vi "Process.vi"(8 "error in":errorcluster, 11 "Example Instrument UI":refnum<class "ExampleInstrument.UI.lvclass">) -> (0 "error out":errorcluster, 3 "Example Instrument UI out":refnum<class "ExampleInstrument.UI.lvclass">)   [LabVIEW 2016, in "ExampleInstrument.UI.lvclass"]
doc: "---------------------------------------------------------------\nJKI State Machine Objects™\nhttp://jki.net/state-machine-objects/\nCopyright (C) 2005-2015, JKI <info@jki.net>\nALL RIGHTS RESERVEDJKI State Machine Objects (SMO) 1.0.0.5\nJKI - JKI\nCopyright (c) 2016, JKI"
uses:
  ExampleInstrument.UI.lvclass
  C:/Program Files (x86)/National Instruments/LabVIEW 2016/vi.lib/JKI/JKI SMO/SMO/SMO.lvclass
  C:/Program Files (x86)/National Instruments/LabVIEW 2016/vi.lib/JKI/JKI SMO/SMO.UI/SMO.UI.lvclass
  <vilib>/JKI/JKI SMO/SMO/Typedefs/Parent Call--Enum.ctl
  ExampleInstrument.UI.lvclass/ExampleInstrument.UI.ctl
  Example Instrument/Typedefs/ExampleInstrument.getAll--Cluster.ctl
  <vilib>/JKI/JKI SMO/SMO.UI/SMO.UI.lvclass
  lvsrc/SMOs/Instrument/Instrument.lvclass
  <vilib>/JKI/JKI SMO/SMO/SMO.lvclass
  Example Instrument/ExampleInstrument.lvclass
panel:
  out "Numeric":u32
  out "Instrument Response":dbl
  in  "Set Parameter":bool
  in  "Parameter":dbl
  in  "STOP":bool
  out "SMO string":string
  out "SMO Boolean":bool
  out "Logger SMO":dbl
  out "Levy 1":dbl
  # "#todo\nmake UI here. maybe include a nice picture of the hardware?"
  # "#todo\nadd buttons to do stuff (e.g., change a setting)\nButtons should trigger an event"
  # "#todo\nresize this box if you want your UI to be different size"
  # "SMO UI Template"
  # "For instructions on how to use the JKI State Machine Objects, examples and video tutorials, visit:\nhttp://jki.net/state-machine-objects/\n\nJKI State Machine Objects™\nhttp://jki.net/state-machine-objects/\nCopyright (C) 2005-2015, JKI <info@jki.net>\nALL RIGHTS RESERVED"
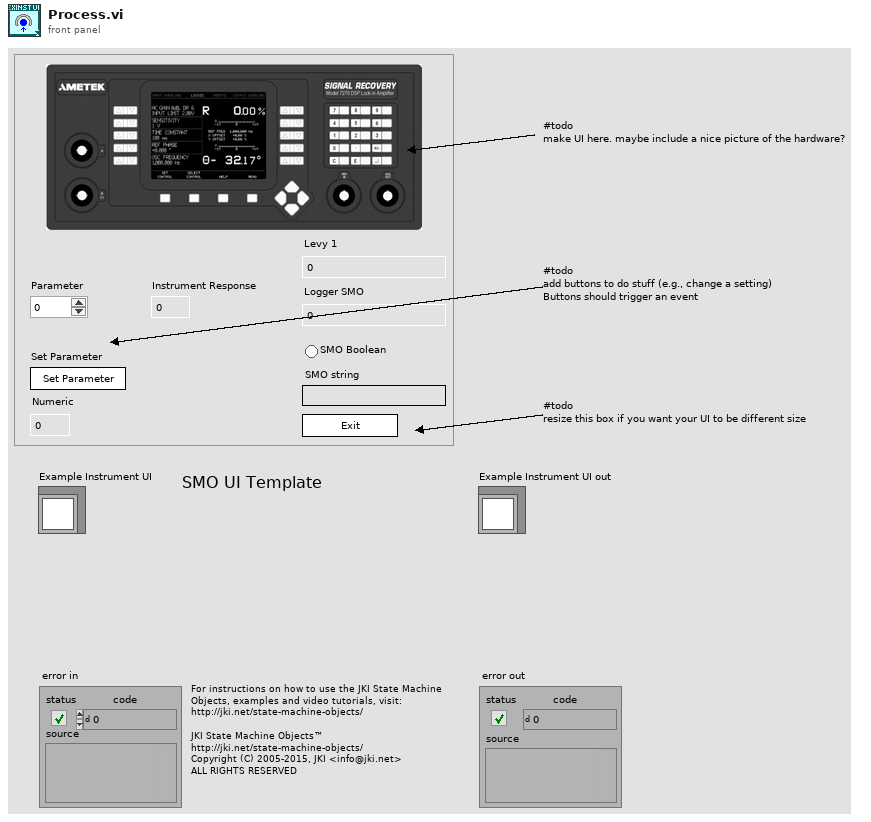
[diagram p1: front panel]
types:
  T1 = typedef "SMO.lvclass/Parent Call--Enum.ctl" = enum16{"Allows parent to run", "Does not request parent to run"}
  T2 = enum32{"invalid app kind", "Development System", "Run Time System", "Student Edition", "Embedded LabVIEW", "Evaluation", "Custom"}
  T3 = enum32{"Invalid", "Standard", "Closed", "Hidden", "Minimized", "Maximized"}
  T4 = typedef "ExampleInstrument.lvclass/ExampleInstrument.getAll--Cluster.ctl" = cluster{"Levy 1":dbl, "Logger SMO":dbl, "SMO Boolean":bool, "SMO String":string}
  T5 = cluster{"Core":cluster{"Current VI Reference":refnum<vi>, "Close Panel on Exit?":bool, "error":errorcluster}, "Self Reference":refnum<class "ExampleInstrument.UI.lvclass">, "Instrument":refnum<class "Instrument.lvclass">, "getAll":variant, "Parameter":dbl}
  T6 = cluster{"Current VI Reference":refnum<vi>, "Close Panel on Exit?":bool, "error":errorcluster}
  T7 = typedef "SMO.lvclass/Protected Events.ctl" = cluster{"StopProcesses":refnum<user-event>, "AbortProcesses":refnum<user-event>, "Config Changed":refnum<user-event>, "Dependency":refnum<user-event>}
  T8 = typedef "Instrument.lvclass/PublicEvents--Cluster.ctl" = cluster{"MessageFromProcess":refnum<user-event>}
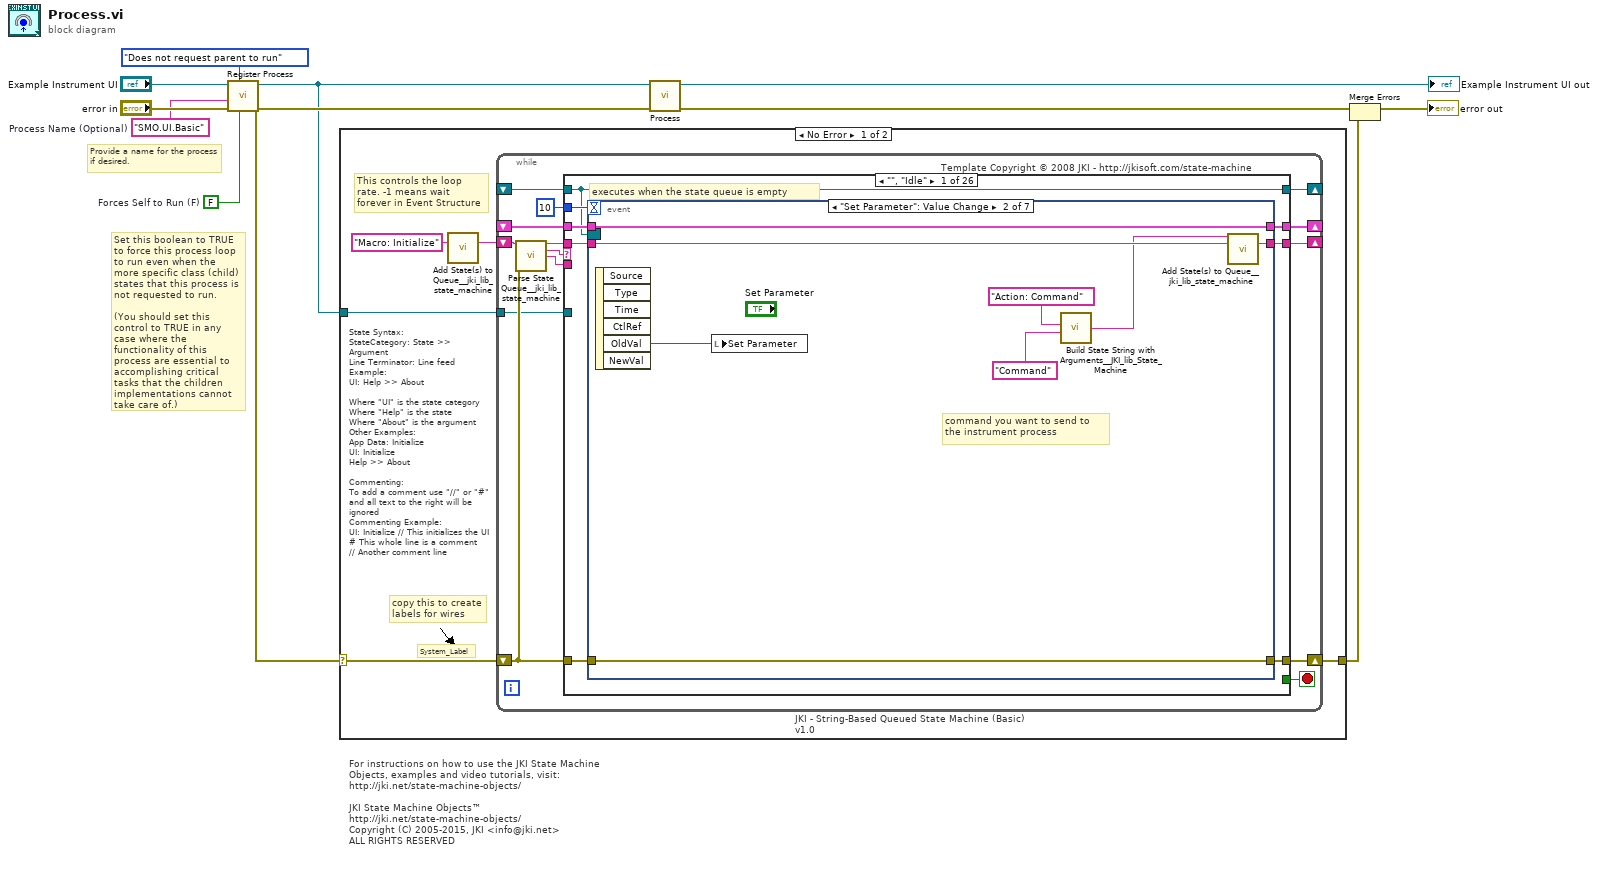
[diagram p0: block diagram]
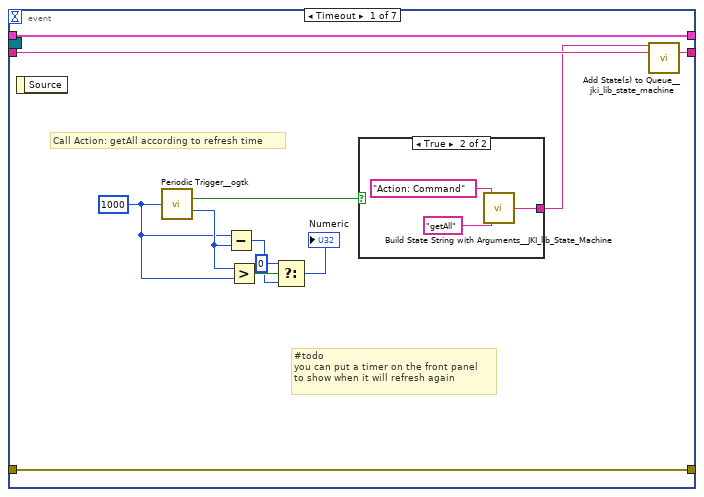
[diagram p2: hidden frame]
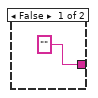
[diagram p3: hidden frame]
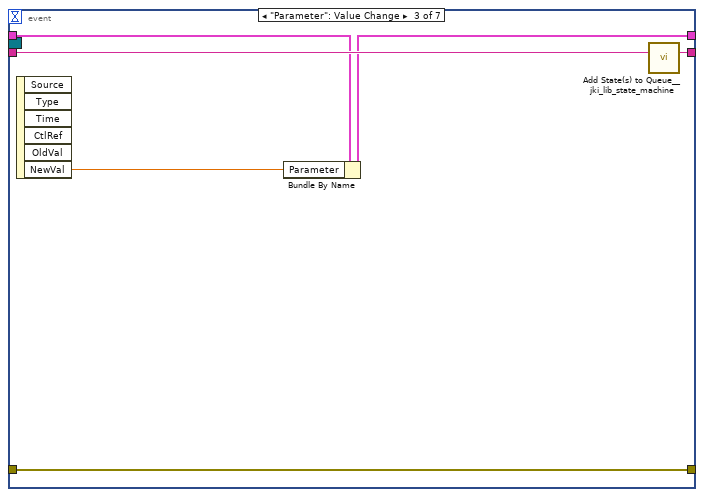
[diagram p4: hidden frame]
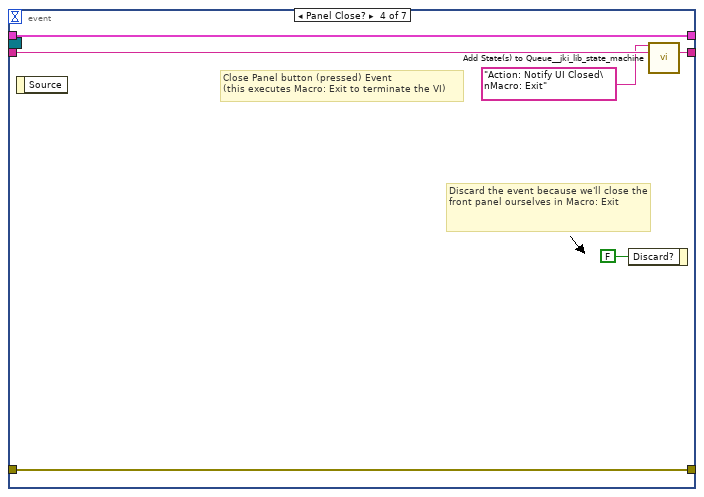
[diagram p5: hidden frame]
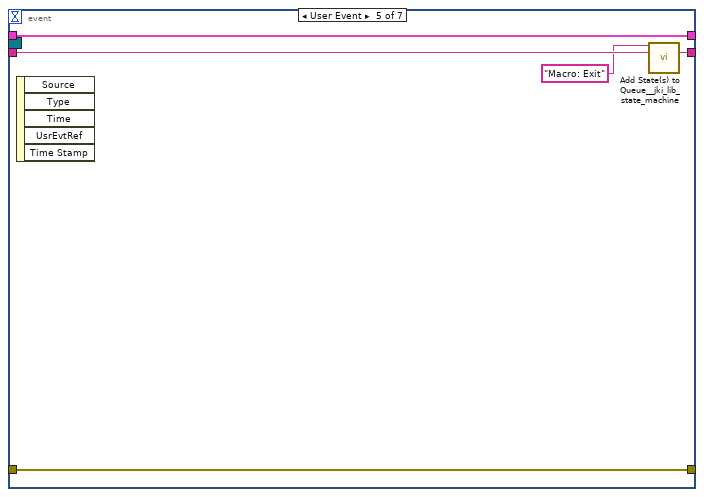
[diagram p6: hidden frame]
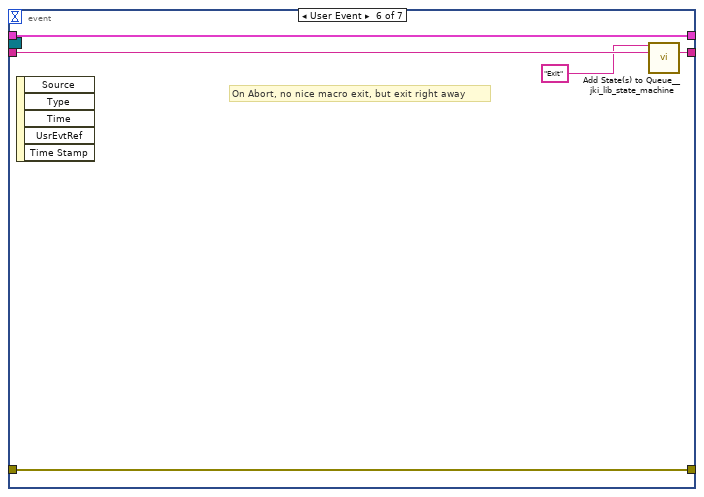
[diagram p7: hidden frame]
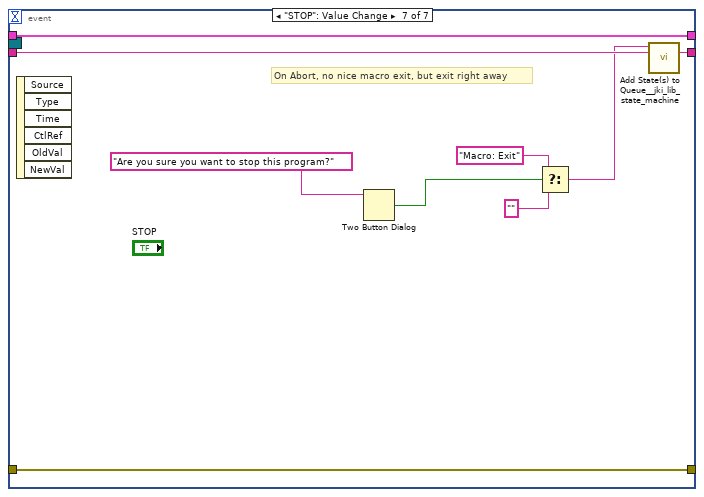
[diagram p8: hidden frame]
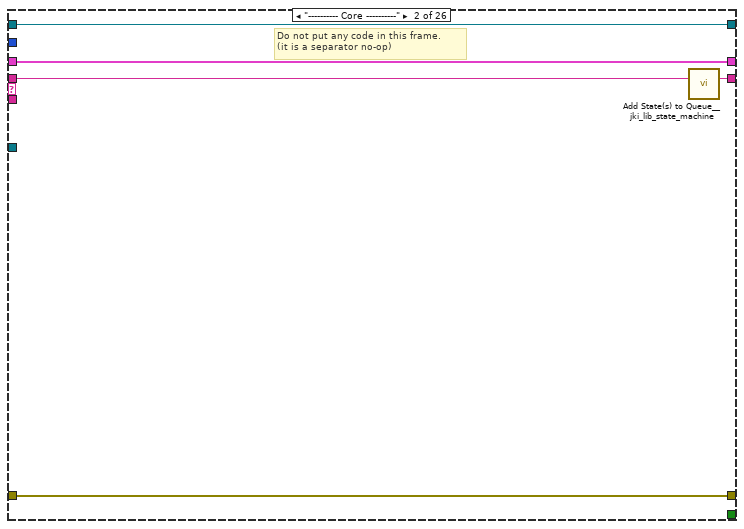
[diagram p9: hidden frame]
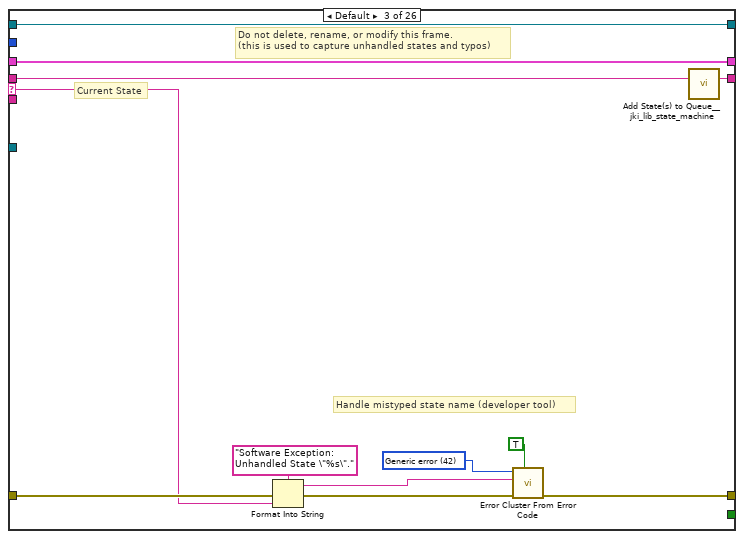
[diagram p10: hidden frame]
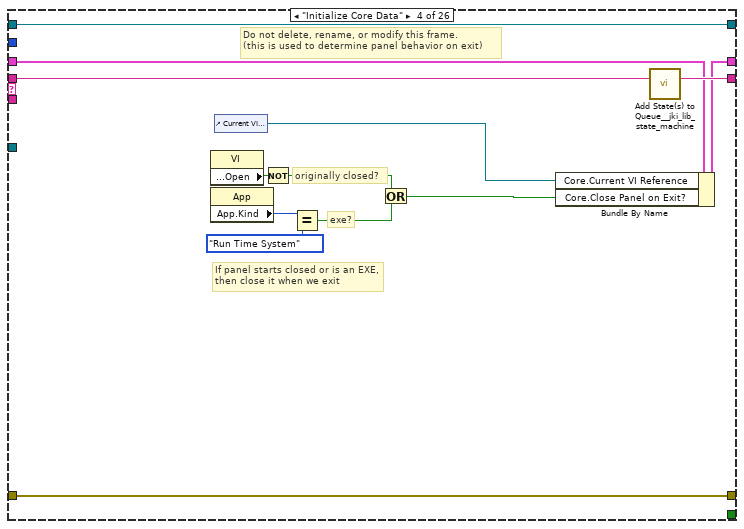
[diagram p11: hidden frame]
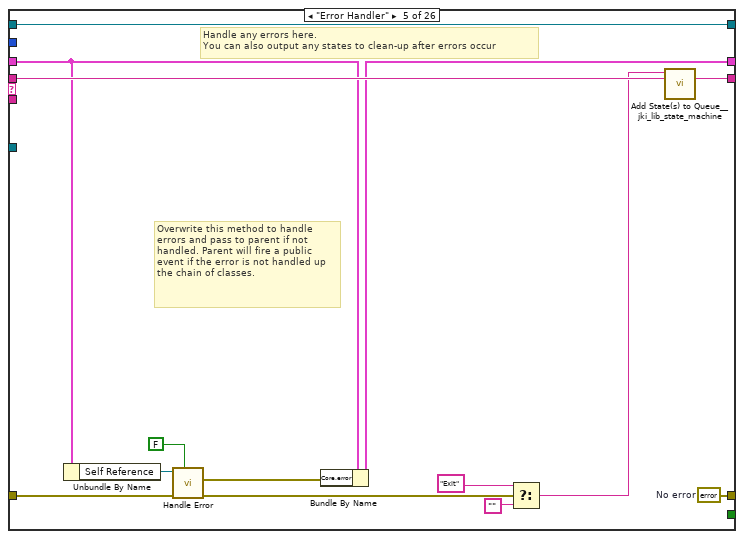
[diagram p12: hidden frame]
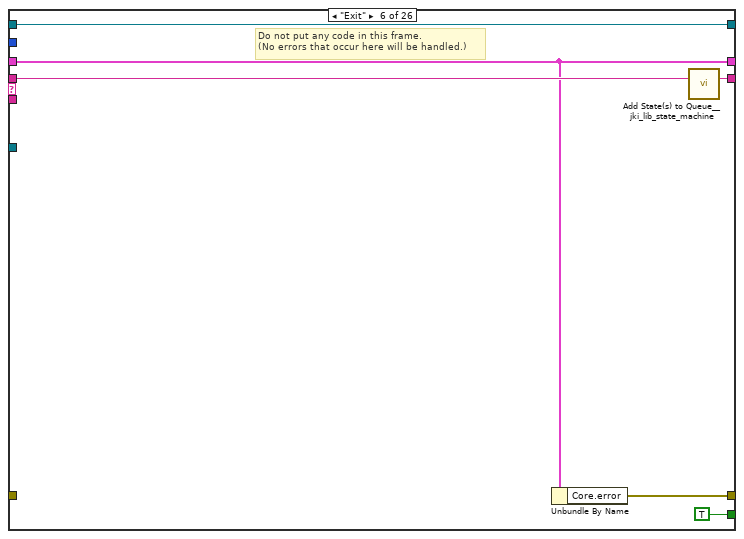
[diagram p13: hidden frame]
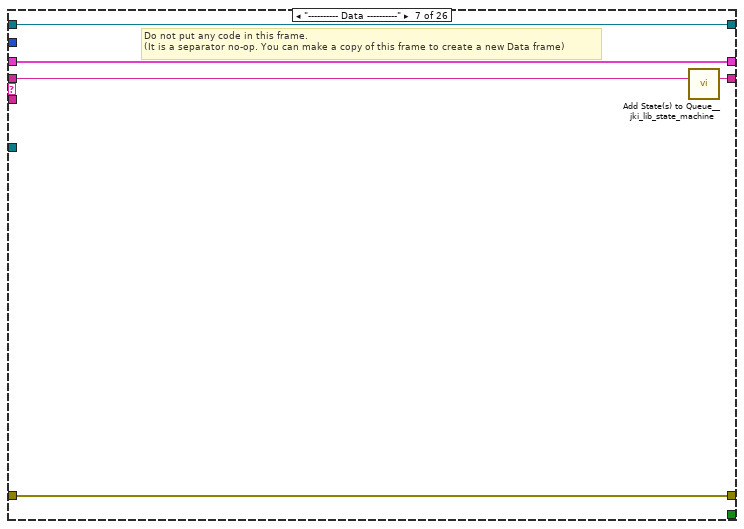
[diagram p14: hidden frame]
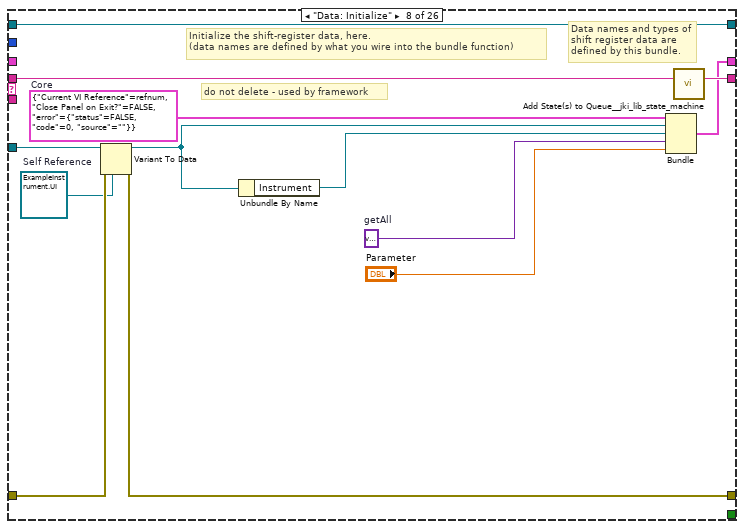
[diagram p15: hidden frame]
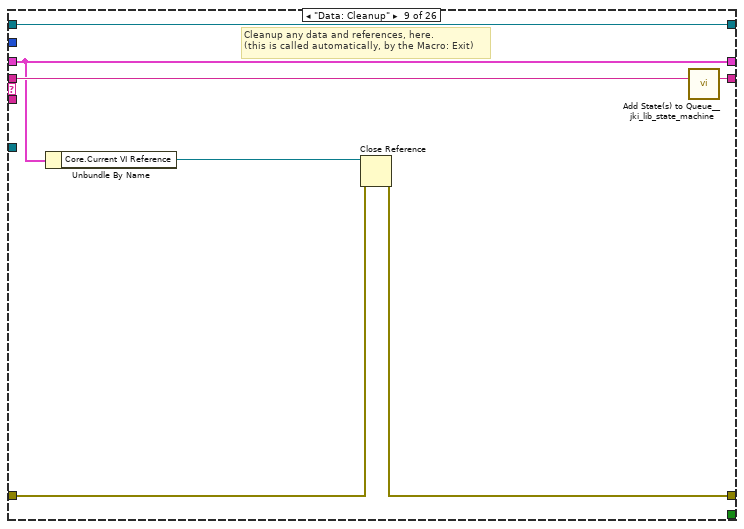
[diagram p16: hidden frame]
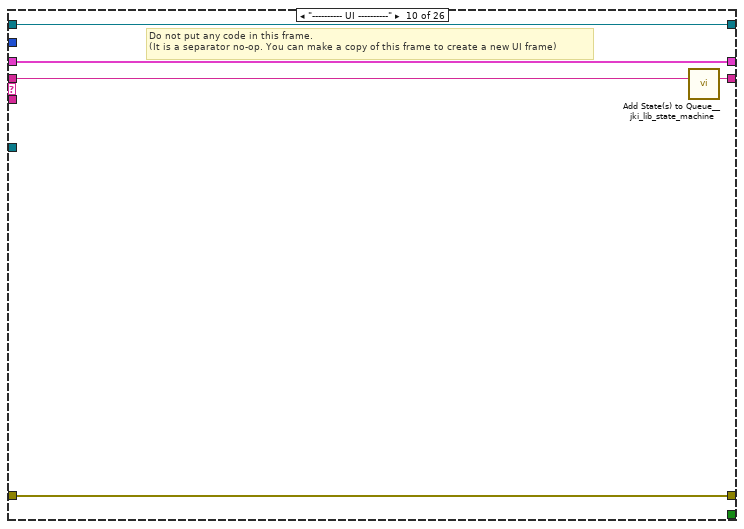
[diagram p17: hidden frame]
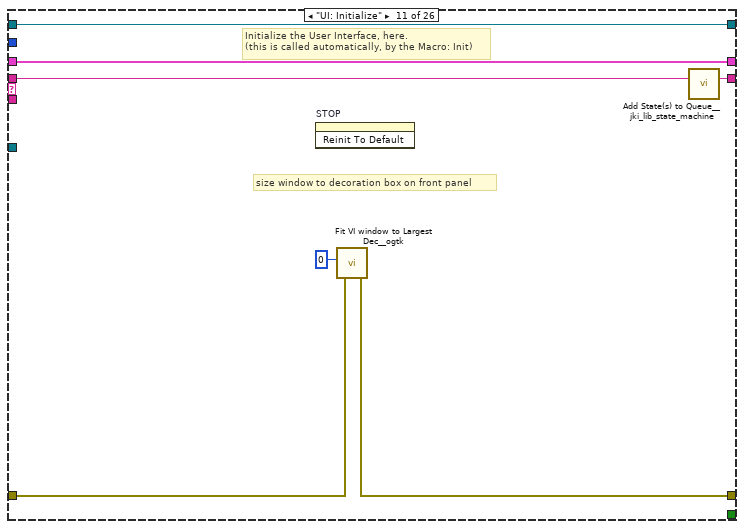
[diagram p18: hidden frame]
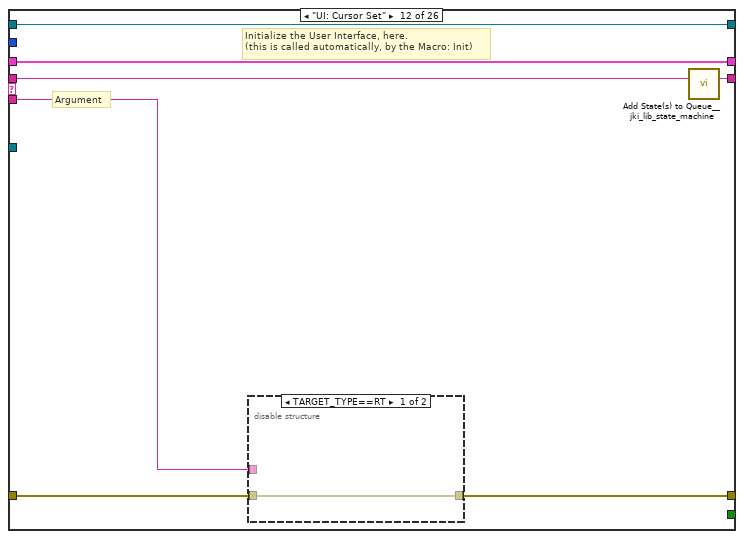
[diagram p19: hidden frame]
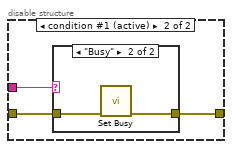
[diagram p20: hidden frame]
diagram:
  w2 = FALSE  # Forces Self to Run (F)
  w1 = "SMO.UI.Basic"  # Process Name (Optional)
  # "Provide a name for the process\nif desired."
  # "Set this boolean to TRUE to force this process loop to run even when the more specific class (child) states that this process is not requested to run.\n\n(You should set this control to TRUE in any case where the functionality of this process are essential to accomplishing critical tasks that the children implementations cannot take care of.)"
  # "For instructions on how to use the JKI State Machine Objects, examples and video tutorials, visit:\nhttp://jki.net/state-machine-objects/\n\nJKI State Machine Objects™\nhttp://jki.net/state-machine-objects/\nCopyright (C) 2005-2015, JKI <info@jki.net>\nALL RIGHTS RESERVED"
  n1 = call <vilib>:"Register Process.vi"("Forces Self to Run (F)"=w2, "Parent Call"=Parent_Call--Enum."Does not request parent to run", "error in (no error)"="error in", "Process Name (optional)"=w1, "SMO"="Example Instrument UI") -> ("error out"=w8:errorcluster, "SMO out"=w7:refnum<class "ExampleInstrument.UI.lvclass">)  [unwired: 5 in]
  n2 = case shown="No Error" w8 {
    selector: w8 -> [w13 w371]
    tunnel: w7 -> [w14 _]
    tunnel: [w12 w371] -> w4
    frame No Error {
      # "State Syntax:\nStateCategory: State >> Argument\nLine Terminator: Line feed\nExample:\nUI: Help >> About\n\nWhere \"UI\" is the state category\nWhere \"Help\" is the state\nWhere \"About\" is the argument\nOther Examples:\nApp Data: Initialize\nUI: Initialize\nHelp >> About\n\nCommenting:\nTo add a comment use \"//\" or \"#\" and all text to the right will be ignored\nCommenting Example:\nUI: Initialize // This initializes the UI\n# This whole line is a comment\n// Another comment line"
      # "copy this to create labels for wires"
      # "This controls the loop rate. -1 means wait forever in Event Structure"
      # "System_Label"
      n3 = call <vilib>:"Add State(s) to Queue__jki_lib_state_machine.vi"("State(s) in (\"\")"="Macro: Initialize") -> ("States Out"=w16:string)  [unwired: 14 in]
      n4 = while "JKI - String-Based Queued State Machine (Basic) v1.0" {
        shift-right: [w23] -> _
        shift-left: _ -> [w22]
        shift-right: [w26] -> w12
        shift-left: w13 -> [w20]
        shift-right: [w25] -> _
        shift-left: w16 -> [w27]
        tunnel: w14 -> [w19]
        shift-right: [w18] -> _
        shift-left: _ -> [w17]
        stop <- w24 stop-if-true
        # "Template Copyright © 2008 JKI - http://jkisoft.com/state-machine"
        n5 = call <vilib>:"Parse State Queue__jki_lib_state_machine.vi"("State Queue"=w27, "Error In (no error)"=w20) -> ("Remaining States"=w29:string, "Current State"=w30:string, "Arguments"=w28:string)  [unwired: 11 in]
        n6 = case shown="\"\", \"Idle\"" w30 {
          selector: w30 -> [_ _ w100 _ _ _ _ _ _ _ _ _ _ _ _ _ _ _ _ _ _ _ _ _ _ _]
          tunnel: w29 -> [w38 w98 w104 w123 w137 w143 w148 w161 w168 w173 w180 w187 w203 w235 w244 w258 w263 w274 w281 w286 w299 w305 w312 w319 w332 w351]
          tunnel: w28 -> [_ _ _ _ _ _ _ _ _ _ _ w181 w197 _ _ _ _ _ _ _ _ _ _ _ _ w339]
          tunnel: w22 -> [w36 w95 w102 w114 w126 w139 w145 _ w163 w170 w178 w185 w199 w232 w240 w249 w260 w271 w276 w283 w297 w303 w308 w315 w329 w348]
          tunnel: [w35 w96 w106 w120 w128 w138 w146 w157 w164 w171 w175 w182 w200 w233 w242 w256 w261 w265 w277 w284 w292 w300 w309 w313 w325 w341] -> w26
          tunnel: w20 -> [w34 w96 w105 w120 w133 _ w146 w158 w165 w171 w176 w183 w201 w233 w242 w256 w261 w266 w278 w284 w294 w301 w309 w314 w326 w342]
          tunnel: [w37 w97 w103 w122 w136 w142 w147 w160 w167 w172 w179 w186 w202 w234 w243 w257 w262 w273 w280 w285 w298 w304 w311 w318 w331 w350] -> w25
          tunnel: [_ _ _ _ _ TRUE _ _ _ _ _ _ _ _ _ _ _ _ _ _ _ _ _ _ _ _] -> w24
          tunnel: [w33 w95 w102 w121 w125 w139 w145 w159 w163 w170 w178 w185 w199 w232 w240 w249 w260 w271 w276 w283 w297 w303 w307 w315 w329 w345] -> w23
          tunnel: 10 ("Timeout") -> [w32 _ _ _ _ _ _ _ _ _ _ _ _ _ _ _ _ _ _ _ _ _ _ _ _ _]
          tunnel: w19 -> [_ _ _ _ _ _ _ w155 _ _ _ _ _ _ _ _ _ _ _ _ _ _ _ _ _ _]
          tunnel: [w31 w94 w99 w111 w135 w140 w144 w154 w162 w169 w177 w184 w196 w231 w241 w250 w259 w272 w279 w282 w296 w302 w310 w317 w330 w349] -> w18
          tunnel: w17 -> [w31 w94 w99 w111 w135 w140 w144 w154 w162 w169 w177 w184 w196 w231 w241 w250 w259 w272 w279 w282 _ w302 w310 w317 w330 w349]
          frame "", "Idle" {
            # "executes when the state queue is empty"
            n7 = event shown="[1] \"Set Parameter\": Value Change" {
              selector: w31 -> [_ _ _ _ _ _ _]
              dyn-events: _ -> [_ _ _ _ _ _ _]
              timeout: w32 -> [_ _ _ _ _ _ _]
              tunnel: w38 -> [w50 w62 w68 w74 w79 w84 w93]
              tunnel: [w49 w61 w67 w73 w78 w83 w92] -> w37
              tunnel: w36 -> [w47 w59 w64 w70 w76 w81 w90]
              tunnel: [w48 w60 w66 w69 w77 w82 w91] -> w35
              tunnel: w34 -> [w48 w60 w66 w69 w77 w82 w91]
              tunnel: [w47 w59 w63 w70 w76 w81 w90] -> w33
              event Timeout {
                w43 = u32 1000 ("time (ms)")
                # "#todo\nyou can put a timer on the front panel\nto show when it will refresh again"
                # "Call Action: getAll according to refresh time"
                n8 = event-data() -> ()  [unwired: 1 in, 1 out]
                n9 = call <userlib>:"Periodic Trigger__ogtk.vi"("time (ms)"=w43) -> ("Triggered"=w45:bool, "timer value"=w44:u32)  [unwired: 12 in, 1 out]
                n10 = Subtract(x=w43, y=w44) -> (x-y=w40:u32)
                n11 = Greater?(x=w44, y=w43) -> (0:w42:bool)
                n12 = Select(t=u32 0, s=w42, f=w40) -> (s? t:f=→"Numeric":u32)
                n13 = case shown="True" w45 {
                  tunnel: ["" ("State(s) in Front (\"\")") w52] -> w46
                  frame False {
                  }
                  frame True {
                    n14 = call <vilib>:"Build State String with Arguments__JKI_lib_State_Machine.vi"("Arguments (\"\")"="getAll" ("State(s) in Front (\"\")"), "State"="Action: Command" ("State(s) in Front (\"\")")) -> ("State with Arguments"=w52:string)  [unwired: 4 in]
                  }
                }
                n15 = call <vilib>:"Add State(s) to Queue__jki_lib_state_machine.vi"("State(s) in Front (\"\")"=w46, "State(s) in (\"\")"=w50) -> ("States Out"=w49:string)  [unwired: 13 in]
              }
              event "Set Parameter": Value Change {
                # "command you want to send to\nthe instrument process"
                n16 = event-data() -> ("OldVal"=w58:bool)  [unwired: 1 in, 5 out]
                n17 = local write "Set Parameter"(w58) -> ()
                n18 = call <vilib>:"Build State String with Arguments__JKI_lib_State_Machine.vi"("Arguments (\"\")"="Command" ("State(s) in Front (\"\")"), "State"="Action: Command" ("State(s) in Front (\"\")")) -> ("State with Arguments"=w55:string)  [unwired: 4 in]
                n19 = call <vilib>:"Add State(s) to Queue__jki_lib_state_machine.vi"("State(s) in Front (\"\")"=w55, "State(s) in (\"\")"=w62) -> ("States Out"=w61:string)  [unwired: 13 in]
              }
              event "Parameter": Value Change {
                n20 = event-data() -> ("NewVal"=w65:dbl)  [unwired: 1 in, 5 out]
                n21 = Bundle By Name(cluster=w64, "Parameter"=w65) -> (w63:T5)
                n22 = call <vilib>:"Add State(s) to Queue__jki_lib_state_machine.vi"("State(s) in (\"\")"=w68) -> ("States Out"=w67:string)  [unwired: 14 in]
              }
              event Panel Close? {
                # "Discard the event because we'll close the front panel ourselves in Macro: Exit"
                # "Close Panel button (pressed) Event\n(this executes Macro: Exit to terminate the VI)"
                n23 = event-data() -> ()  [unwired: 1 in, 1 out]
                n24 = event-data("Discard?"=FALSE) -> ()  [unwired: 1 in, 1 out]
                n25 = call <vilib>:"Add State(s) to Queue__jki_lib_state_machine.vi"("State(s) in Front (\"\")"="Action: Notify UI Closed\nMacro: Exit", "State(s) in (\"\")"=w74) -> ("States Out"=w73:string)  [unwired: 13 in]
              }
              event User Event {
                n26 = event-data() -> ()  [unwired: 1 in, 5 out]
                n27 = call <vilib>:"Add State(s) to Queue__jki_lib_state_machine.vi"("State(s) in Front (\"\")"="Macro: Exit", "State(s) in (\"\")"=w79) -> ("States Out"=w78:string)  [unwired: 13 in]
              }
              event User Event {
                # "On Abort, no nice macro exit, but exit right away"
                n28 = event-data() -> ()  [unwired: 1 in, 5 out]
                n29 = call <vilib>:"Add State(s) to Queue__jki_lib_state_machine.vi"("State(s) in Front (\"\")"="Exit", "State(s) in (\"\")"=w84) -> ("States Out"=w83:string)  [unwired: 13 in]
              }
              event "STOP": Value Change {
                # "On Abort, no nice macro exit, but exit right away"
                n30 = event-data() -> ()  [unwired: 1 in, 6 out]
                n31 = Two Button Dialog(message="Are you sure you want to stop this program?") -> (T button?=w89:bool)  [unwired: 2 in]
                n32 = Select(t="Macro: Exit", s=w89, f="") -> (s? t:f=w85:string)
                n33 = call <vilib>:"Add State(s) to Queue__jki_lib_state_machine.vi"("State(s) in Front (\"\")"=w85, "State(s) in (\"\")"=w93) -> ("States Out"=w92:string)  [unwired: 13 in]
              }
            }
          }
          frame "---------- Core ----------" {
            # "Do not put any code in this frame.\n(it is a separator no-op)"
            n34 = call <vilib>:"Add State(s) to Queue__jki_lib_state_machine.vi"("State(s) in (\"\")"=w98) -> ("States Out"=w97:string)  [unwired: 14 in]
          }
          frame Default {
            w109 = 42 items=["No error", "Argument error", "Memory is full", "Out of zone", "End of file", "File already open", "Generic file I/O error", "File not found", "File permission error", "Disk is full", "Duplicate path", "Too many files open", "System feature not enabled", "Resource file not found", "Cannot add resource", "Resource not found", "Image not found", "Image memory error", "Pen does not exist", "Config type invalid", "Config token not found", "Config parse error", "Config memory error", "Bad external code format", "Bad external code offset", "External code not present", "Null window", "Destroy window error", "Null menu", "Print aborted", "Bad print record", "Print driver error", "Windows error during printing", "Memory error during printing", "Print dialog error", "Generic print error", "Invalid device refnum", "Device not found", "Device parameter error", "Device unit error", "Cannot open device", "Device call aborted", "Generic error", "Cancelled by user", "Object ID too low", "Object ID too high", "Object not in heap", "Unknown heap", "Unknown object (invalid DefProc)", "Unknown object (DefProc not in table)", "Message out of range", "Invalid (null) method", "Unknown message", "Manager call not supported", "Bad address", "Network operation in progress", "Network operation timed out", "Connection is busy", "Network attribute not supported", "Network error", "Address in use", "System out of memory", "Connection aborted", "Connection refused", "Not connected", "Already connected", "Connection closed", "Initialization error (interapplication manager)", "Bad occurrence", "Wait on unbound occurrence handler", "Occurrence queue overflow", "Datalog type conflict", "Unused", "Unrecognized type (interapplication manager)", "Memory corrupt", "Failed to make temporary DLL", "Old CIN version", "Drag socket not found", "Failed to load drop-object", "Failed to register OLE object", "Failed to release OLE object", "Format specifier type mismatch", "Unknown format specifier", "Too few format specifiers", "Too many format specifiers", "Scan failed", "Newer CIN version", "Error converting to variant", "Runtime menu error", "Password tampered", "Variant attribute not found", "Incompatible variant data type", "Event data is not available", "Event Store is not present", "Occurrence is not found", "Event Queue is not created", "Event info is not available", "Refnum passed is NULL", "Error retrieving Class GUID", "Error retrieving CoClass GUID", "Error retrieving TypeLib GUID.", "Bad built application magic bytes.", "Specific driver is different from the specific driver associated with the Logical Name.", "There is no session opened to the class driver.", "Max Error", "MAX - Error with config objects", "MAX - Error loading configuration", "MAX - Group not supported"]
            # "Current State"
            # "Do not delete, rename, or modify this frame.\n(this is used to capture unhandled states and typos)"
            # "Handle mistyped state name (developer tool)"
            n35 = Format Into String(format string="Software Exception: Unhandled State \"%s\"." ("message"), error in=w105, w100) -> (resulting string=w108:string, error out=w107:errorcluster)  [unwired: 1 in]
            n36 = call <vilib>:"Error Cluster From Error Code.vi"("show call chain? (False)"=TRUE, "error in (no error)"=w107, "error message (\"\")"=w108, "error code (0)"=w109) -> ("error out"=w106:errorcluster)  [unwired: 5 in]
            n37 = call <vilib>:"Add State(s) to Queue__jki_lib_state_machine.vi"("State(s) in (\"\")"=w104) -> ("States Out"=w103:string)  [unwired: 14 in]
          }
          frame "Initialize Core Data" {
            # "Do not delete, rename, or modify this frame.\n(this is used to determine panel behavior on exit)"
            # "originally closed?"
            # "exe?"
            # "If panel starts closed or is an EXE, then close it when we exit"
            n38 = property class="VI"() -> ("Front Panel.Open"=w119:bool)  [unwired: 2 in, 2 out]
            n39 = property class="App"() -> ("App.Kind"=w118:T2)  [unwired: 2 in, 2 out]
            n40 = control-ref of="Current VI Reference"() -> (w112:refnum<vi>)
            n41 = Not(x=w119) -> (.not. x?=w116:bool)
            n42 = Equal?(x=w118, y=T2."Run Time System" ("Application:Kind")) -> (x = y?=w115:bool)
            n43 = Or(x=w116, y=w115) -> (x .or. y?=w113:bool)
            n44 = Bundle By Name(cluster=w114, "Core.Current VI Reference"=w112, "Core.Close Panel on Exit?"=w113) -> (w121:T5)
            n45 = call <vilib>:"Add State(s) to Queue__jki_lib_state_machine.vi"("State(s) in (\"\")"=w123) -> ("States Out"=w122:string)  [unwired: 14 in]
          }
          frame "Error Handler" {
            w128 = errorcluster {"status"=FALSE, "code"=0, "source"=""}  # No error
            # "Overwrite this method to handle errors and pass to parent if not handled. Parent will fire a public event if the error is not handled up the chain of classes."
            # "Handle any errors here.\nYou can also output any states to clean-up after errors occur"
            n46 = Unbundle By Name(w126) -> ("Self Reference"=w134:refnum<class "ExampleInstrument.UI.lvclass">)
            n47 = call-dynamic "Handle Error.vi"("Stop on Unhandled Error (T)"=FALSE, "error in"=w133, "SMO"=w134) -> ("handling error"=w129:errorcluster, "Unhandled error"=w127:errorcluster)  [unwired: 6 in, 1 out]
            n48 = Bundle By Name(cluster=w126, "Core.error"=w127) -> (w125:T5)
            n49 = Select(t="Exit", s=w129, f="") -> (s? t:f=w130:string)
            n50 = call <vilib>:"Add State(s) to Queue__jki_lib_state_machine.vi"("State(s) in Front (\"\")"=w130, "State(s) in (\"\")"=w137) -> ("States Out"=w136:string)  [unwired: 13 in]
          }
          frame "Exit" {
            # "Do not put any code in this frame.\n(No errors that occur here will be handled.)"
            n51 = Unbundle By Name(w139) -> ("Core.error"=w138:errorcluster)
            n52 = call <vilib>:"Add State(s) to Queue__jki_lib_state_machine.vi"("State(s) in (\"\")"=w143) -> ("States Out"=w142:string)  [unwired: 14 in]
          }
          frame "---------- Data ----------" {
            # "Do not put any code in this frame.\n(It is a separator no-op. You can make a copy of this frame to create a new Data frame)"
            n53 = call <vilib>:"Add State(s) to Queue__jki_lib_state_machine.vi"("State(s) in (\"\")"=w148) -> ("States Out"=w147:string)  [unwired: 14 in]
          }
          frame "Data: Initialize" {
            w150 = variant  # getAll
            w153 = T6 {"Current VI Reference"=refnum, "Close Panel on Exit?"=FALSE, "error"={"status"=FALSE, "code"=0, "source"=""}}  # Core
            w156 = refnum<class "ExampleInstrument.UI.lvclass"> refnum  # Self Reference
            # "do not delete - used by framework"
            # "Data names and types of shift register data are defined by this bundle."
            # "Initialize the shift-register data, here.\n(data names are defined by what you wire into the bundle function)"
            n54 = Variant To Data(error in=w158, type=w156, Variant=w155) -> (data=w152:refnum<class "ExampleInstrument.UI.lvclass">, error out=w157:errorcluster)
            n55 = Unbundle By Name(w152) -> ("Instrument"=w151:refnum<class "Instrument.lvclass">)
            n56 = Bundle("Core"=w153, "Self Reference"=w152, "Instrument"=w151, "getAll"=w150, "Parameter"="Parameter") -> (w159:T5)  [unwired: 1 in]
            n57 = call <vilib>:"Add State(s) to Queue__jki_lib_state_machine.vi"("State(s) in (\"\")"=w161) -> ("States Out"=w160:string)  [unwired: 14 in]
          }
          frame "Data: Cleanup" {
            # "Cleanup any data and references, here.\n(this is called automatically, by the Macro: Exit)"
            n58 = Unbundle By Name(w163) -> ("Core.Current VI Reference"=w166:refnum<vi>)
            n59 = Close Reference(reference=w166, error in (no error)=w165) -> (error out=w164:errorcluster)
            n60 = call <vilib>:"Add State(s) to Queue__jki_lib_state_machine.vi"("State(s) in (\"\")"=w168) -> ("States Out"=w167:string)  [unwired: 14 in]
          }
          frame "---------- UI ----------" {
            # "Do not put any code in this frame.\n(It is a separator no-op. You can make a copy of this frame to create a new UI frame)"
            n61 = call <vilib>:"Add State(s) to Queue__jki_lib_state_machine.vi"("State(s) in (\"\")"=w173) -> ("States Out"=w172:string)  [unwired: 14 in]
          }
          frame "UI: Initialize" {
            # "size window to decoration box on front panel"
            # "Initialize the User Interface, here.\n(this is called automatically, by the Macro: Init)"
            n62 = invoke on="STOP" class="Bool (strict)" method="Reinit To Default"() -> ()  [unwired: 3 in, 3 out]
            n63 = call <userlib>:"Fit VI window to Largest Dec__ogtk.vi"("error in (no error)"=w176, "border spacing (2 px)"=0) -> ("error out"=w175:errorcluster)  [unwired: 4 in, 1 out]
            n64 = call <vilib>:"Add State(s) to Queue__jki_lib_state_machine.vi"("State(s) in (\"\")"=w180) -> ("States Out"=w179:string)  [unwired: 14 in]
          }
          frame "UI: Cursor Set" {
            # "Argument"
            # "Initialize the User Interface, here.\n(this is called automatically, by the Macro: Init)"
            n65 = disable-structure shown="TARGET_TYPE==RT" {
              disable-tunnel: w183 -> [w188 w191]
              disable-tunnel: [w188 w190] -> w182
              disable-tunnel: w181 -> [_ w189]
              frame condition #0 {
              }
              frame condition #1 (active) {
                n66 = case shown="\"Busy\"" w189 {
                  tunnel: w191 -> [w193 w195]
                  tunnel: [w192 w194] -> w190
                  frame "Idle", Default {
                    n67 = call <vilib>:"Unset Busy.vi"("error in (no error)"=w193) -> ("error out"=w192:errorcluster)  [unwired: 10 in]
                  }
                  frame "Busy" {
                    n68 = call <vilib>:"Set Busy.vi"("error in (no error)"=w195) -> ("error out"=w194:errorcluster)  [unwired: 9 in, 1 out]
                  }
                }
              }
            }
            n69 = call <vilib>:"Add State(s) to Queue__jki_lib_state_machine.vi"("State(s) in (\"\")"=w187) -> ("States Out"=w186:string)  [unwired: 14 in]
          }
          frame "UI: Front Panel State" {
            # "Argument"
            # "Set Front Panel Open or Closed\n(Usage: \"UI: Front Panel State >> Open|Close\")"
            n70 = Unbundle By Name(w199) -> ("Core.Current VI Reference"=w198:refnum<vi>)
            n71 = disable-structure shown="Default" {
              disable-tunnel: w201 -> [w207 w230]
              disable-tunnel: [w206 w230] -> w200
              disable-tunnel: w198 -> [w205 _]
              disable-tunnel: w197 -> [w204 _]
              frame condition #0 (active) {
                n72 = case shown="\"Close\"" w204 {
                  tunnel: w207 -> [w211 w224]
                  tunnel: [w213 w225] -> w206
                  tunnel: w205 -> [w212 w222]
                  frame "Open", Default {
                    n73 = property class="VI"(reference=w212, error in=w211) -> (reference out=w209:refnum<vi>, error out=w210:errorcluster, "FP.State"=w208:T3)
                    n74 = case shown="\"Closed\"" w208 {
                      tunnel: [w216 w219] -> w213
                      tunnel: w210 -> [w215 w219]
                      tunnel: w209 -> [w214 _]
                      frame "Closed" {
                        n75 = invoke class="VI" method="FP.Open"(reference=w214, error in=w215, "Activate"=TRUE, "State"=T3."Standard") -> (error out=w216:errorcluster)  [unwired: 1 in, 4 out]
                      }
                      frame Default {
                      }
                    }
                  }
                  frame "Close" {
                    n76 = property class="VI"(reference=w222, error in=w224) -> (reference out=w221:refnum<vi>, error out=w223:errorcluster, "FP.State"=w220:T3)
                    n77 = case shown="Default" w220 {
                      tunnel: [w226 w229] -> w225
                      tunnel: w223 -> [w226 w228]
                      tunnel: w221 -> [_ w227]
                      frame "Invalid", "Closed" {
                      }
                      frame Default {
                        n78 = invoke class="VI" method="FP.Close"(reference=w227, error in=w228) -> (error out=w229:errorcluster)  [unwired: 1 in, 2 out]
                      }
                    }
                  }
                }
              }
              frame condition #1 {
              }
            }
            n79 = call <vilib>:"Add State(s) to Queue__jki_lib_state_machine.vi"("State(s) in (\"\")"=w203) -> ("States Out"=w202:string)  [unwired: 14 in]
          }
          frame "---------- Macro ----------" {
            # "Do not put any code in this frame.\n(It is a separator no-op. You can make a copy of this frame to create a new Macro frame)"
            n80 = call <vilib>:"Add State(s) to Queue__jki_lib_state_machine.vi"("State(s) in (\"\")"=w235) -> ("States Out"=w234:string)  [unwired: 14 in]
          }
          frame "Macro: Initialize" {
            w238 = "UI: Initialize\n//UI: Front Panel State >> Open"  # UI: Initialize //UI: Front Panel State >> Open
            # "Initialization Macro\n(This is called once, when the VI starts)"
            n81 = call <vilib>:"Add State(s) to Queue__jki_lib_state_machine.vi"("State(s) in Front (\"\")"="Data: Initialize\nInitialize Core Data\nEvents: Register", "State(s) in (\"\")"="Process: Sync", "State(s) at Back (\"\")"=w238) -> ("States Out"=w237:string)  [unwired: 12 in]
            n82 = call <vilib>:"Add State(s) to Queue__jki_lib_state_machine.vi"("State(s) in Front (\"\")"=w237, "State(s) in (\"\")"=w244) -> ("States Out"=w243:string)  [unwired: 13 in]
          }
          frame "Macro: Exit" {
            # "Exit Macro\n(This is called once, when the VI exits)"
            n83 = Unbundle By Name(w249) -> ("Core.Close Panel on Exit?"=w255:bool)
            n84 = Select(t="//UI: Front Panel State >> Close", s=w255, f="") -> (s? t:f=w252:string)
            n85 = call <vilib>:"Add State(s) to Queue__jki_lib_state_machine.vi"("State(s) in Front (\"\")"="Data: Cleanup\nEvents: Unregister\nProcess: Self Terminate", "State(s) in (\"\")"="Process: Sync", "State(s) at Back (\"\")"="Exit") -> ("States Out"=w246:string)  [unwired: 12 in]
            n86 = call <vilib>:"Add State(s) to Queue__jki_lib_state_machine.vi"("State(s) in (\"\")"=w252, "State(s) at Back (\"\")"=w246) -> ("States Out"=w251:string)  [unwired: 13 in]
            n87 = call <vilib>:"Add State(s) to Queue__jki_lib_state_machine.vi"("State(s) in Front (\"\")"=w251, "State(s) in (\"\")"=w258) -> ("States Out"=w257:string)  [unwired: 13 in]
          }
          frame "---------- Process ----------" {
            # "Template Separator\n(You can make a copy of, or modify, this frame)"
            n88 = call <vilib>:"Add State(s) to Queue__jki_lib_state_machine.vi"("State(s) in (\"\")"=w263) -> ("States Out"=w262:string)  [unwired: 14 in]
          }
          frame "Process: Sync" {
            n89 = Unbundle By Name(w271) -> ("Self Reference"=w267:refnum<class "ExampleInstrument.UI.lvclass">)
            n90 = call <vilib>:"WaitOnProcessSync.vi"("error in (no error)"=w266, "SMO"=w267) -> ("error out"=w265:errorcluster, "Don't run?"=w270:bool)  [unwired: 7 in, 1 out]
            n91 = Select(t="Data: Cleanup\nEvents: Unregister\nExit", s=w270, f="") -> (s? t:f=w264:string)
            n92 = call <vilib>:"Add State(s) to Queue__jki_lib_state_machine.vi"("State(s) in Front (\"\")"=w264, "State(s) in (\"\")"=w274) -> ("States Out"=w273:string)  [unwired: 13 in]
          }
          frame "Process: Self Terminate" {
            n93 = Unbundle By Name(w276) -> ("Self Reference"=w275:refnum<class "ExampleInstrument.UI.lvclass">)
            n94 = call <vilib>:"SelfTerminate.vi"("error in (no error)"=w278, "SMO in"=w275) -> ("error out"=w277:errorcluster)  [unwired: 8 in, 1 out]
            n95 = call <vilib>:"Add State(s) to Queue__jki_lib_state_machine.vi"("State(s) in (\"\")"=w281) -> ("States Out"=w280:string)  [unwired: 14 in]
          }
          frame "---------- Events ----------" {
            # "Template Separator\n(You can make a copy of, or modify, this frame)"
            n96 = call <vilib>:"Add State(s) to Queue__jki_lib_state_machine.vi"("State(s) in (\"\")"=w286) -> ("States Out"=w285:string)  [unwired: 14 in]
          }
          frame "Events: Register" {
            # "Expand to add\nmore events"
            # "Base Class Protected Events"
            n97 = Unbundle By Name(w297) -> ("Self Reference"=w290:refnum<class "ExampleInstrument.UI.lvclass">, "Instrument"=w289:refnum<class "Instrument.lvclass">)
            n98 = call <vilib>:"GetProtectedEvents.vi"("SMO"=w290) -> ("error out"=w291:errorcluster, "SMO Protected Events"=w295:T7)  [unwired: 8 in, 1 out]
            n99 = call "Instrument.GetPublicEvents.vi"("Instrument"=w289) -> ("error out"=w287:errorcluster, "Instrument Public Events"=w288:T8)  [unwired: 8 in, 1 out]
            n100 = register-events(w295, w288) -> (reference out=w296:refnum<event-registration>, error out=w293:errorcluster)  [unwired: 2 in]
            n101 = Merge Errors(w287, w294, w293, w291) -> (w292:errorcluster)
            n102 = call <vilib>:"Add State(s) to Queue__jki_lib_state_machine.vi"("State(s) in (\"\")"=w299) -> ("States Out"=w298:string)  [unwired: 14 in]
          }
          frame "Events: Unregister" {
            n103 = Unregister For Events(event registration refnum=w302, error in=w301) -> (error out=w300:errorcluster)
            n104 = call <vilib>:"Add State(s) to Queue__jki_lib_state_machine.vi"("State(s) in (\"\")"=w305) -> ("States Out"=w304:string)  [unwired: 14 in]
          }
          frame "---------- Action ----------" {
            n105 = Unbundle By Name(w308) -> ("Self Reference"=w306:refnum<class "ExampleInstrument.UI.lvclass">)
            n106 = Bundle By Name(cluster=w308, "Self Reference"=w306) -> (w307:T5)
            n107 = call <vilib>:"Add State(s) to Queue__jki_lib_state_machine.vi"("State(s) in (\"\")"=w312) -> ("States Out"=w311:string)  [unwired: 14 in]
          }
          frame "Action: Notify UI Closed" {
            # "Notify that the UI has been closed"
            n108 = Unbundle By Name(w315) -> ("Self Reference"=w316:refnum<class "ExampleInstrument.UI.lvclass">)
            n109 = call <vilib>:"Hide.vi"("error in (no error)"=w314, "SMO.UI"=w316) -> ("error out"=w313:errorcluster)  [unwired: 8 in, 1 out]
            n110 = call <vilib>:"Add State(s) to Queue__jki_lib_state_machine.vi"("State(s) in (\"\")"=w319) -> ("States Out"=w318:string)  [unwired: 14 in]
          }
          frame "Action: Update Front Panel" {
            # "do this way to have nicer UI or only display what you want"
            # "typedef from Child Instrument"
            n111 = Unbundle By Name(w329) -> ("getAll"=w328:variant)
            n112 = Variant To Data(error in=w326, type=T4 {"Levy 1"=0.0, "Logger SMO"=0.0, "SMO Boolean"=FALSE, "SMO String"=""} ("getAll"), Variant=w328) -> (data=w324:T4, error out=w325:errorcluster)
            n113 = Unbundle By Name(w324) -> ("Levy 1"=→"Levy 1":dbl, "Logger SMO"=→"Logger SMO":dbl, "SMO Boolean"=→"SMO Boolean":bool, "SMO String"=→"SMO string":string)
            n114 = call <vilib>:"Add State(s) to Queue__jki_lib_state_machine.vi"("State(s) in (\"\")"=w332) -> ("States Out"=w331:string)  [unwired: 14 in]
          }
          frame "Action: Command" {
            # "#todo:\nconfigure here how to parse messages from Instrument"
            # "command"
            n115 = Unbundle By Name(w348) -> ("Self Reference"=w337:refnum<class "ExampleInstrument.UI.lvclass">, "Instrument"=w335:refnum<class "Instrument.lvclass">, "Parameter"=w344:dbl)
            n116 = call-dynamic "Remote Client.vi"("Wait for Response?"=TRUE, "error in (no error)"=w342, "Data"=w344, "Command"=w339, "Instrument in"=w335) -> ("error out"=w343:errorcluster, "Data out"=w346:variant, "Command out"=w347:string)  [unwired: 3 in, 1 out]
            n117 = case shown="\"getAll\"" w347 {
              tunnel: w346 -> [_ w358 w370]
              tunnel: w343 -> [w356 w361 w368]
              tunnel: [w356 w361 w366] -> w341
              tunnel: [w354 w360 w365] -> w338
              tunnel: w337 -> [w354 w360 w365]
              tunnel: ["" ("State(s) in Front (\"\")") "Action: Update Front Panel" ("State(s) in Front (\"\")") "" ("State(s) in Front (\"\")")] -> w336
              tunnel: w335 -> [w355 w357 w363]
              tunnel: [w355 w357 w363] -> w334
              tunnel: [variant ("Data out") w358 variant ("Data out")] -> w333
              frame Default {
              }
              frame "getAll" {
              }
              frame "setMagnet" {
                n118 = Variant To Data(error in=w368, type=0.0 ("Magnet Return"), Variant=w370) -> (data=→"Instrument Response":dbl, error out=w366:errorcluster)
              }
            }
            n119 = Bundle By Name(cluster=w348, "Self Reference"=w338, "Instrument"=w334, "getAll"=w333) -> (w345:T5)
            n120 = call <vilib>:"Add State(s) to Queue__jki_lib_state_machine.vi"("State(s) in Front (\"\")"=w336, "State(s) in (\"\")"=w351) -> ("States Out"=w350:string)  [unwired: 13 in]
          }
        }
      }
    }
    frame Error {
    }
  }
  n121 = call-parent "Process.vi"("error in (no error)"=w8, "SMO.UI"=w7) -> ("error out"=w5:errorcluster, "SMO.UI out"=→"Example Instrument UI out":refnum<class "ExampleInstrument.UI.lvclass">)  [unwired: 8 in]
  n122 = Merge Errors(w5, w4) -> (→"error out":errorcluster)
